vi "stringtoxml.vi"(1 "String to write":string, 2 "XML Tag":string) -> (0 "xml string":string)   [LabVIEW 2012]
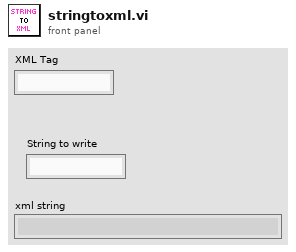
[diagram p1: front panel]
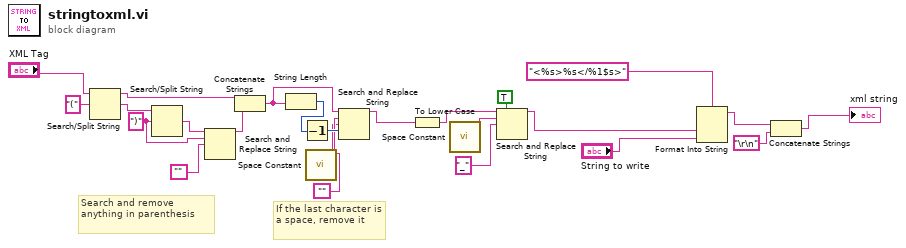
[diagram p0: block diagram]
diagram:
  w9 = ")" ("search string/char (-)")
  # "If the last character is a space, remove it"
  # "Search and remove anything in parenthesis"
  n1 = Search/Split String(string="XML Tag", search string/char (-)="(") -> (substring before match=w12:string, match + rest of string=w13:string)  [unwired: 1 in, 1 out]
  n2 = Search/Split String(string=w13, search string/char (-)=w9) -> (match + rest of string=w11:string)  [unwired: 1 in, 2 out]
  n3 = Search and Replace String(input string=w11, search string=w9, replace string="") -> (result string=w8:string)  [unwired: 5 in, 3 out]
  n4 = Concatenate Strings(w12, w8) -> (w5:string)
  n5 = String Length(string=w5) -> (length=w7:i32)
  n6 = Decrement(x=w7) -> (x-1=w6:i32)
  n7 = call <vilib>:"Space Constant.vi"() -> ("String"=w4:string)
  n8 = Search and Replace String(input string=w5, search string=w4, replace string="", offset=w6) -> (result string=w1:string)  [unwired: 4 in, 3 out]
  n9 = To Lower Case(string=w1) -> (all lower case string=w19:string)
  n10 = call <vilib>:"Space Constant.vi"() -> ("String"=w17:string)
  n11 = Search and Replace String(replace all?=TRUE ("replace all? (F)"), input string=w19, search string=w17, replace string="_") -> (result string=w15:string)  [unwired: 4 in, 3 out]
  n12 = Format Into String(format string="<%s>%s</%1$s>" ("format string (<%s>%d</%1$s>)"), w15, "String to write") -> (resulting string=w22:string)  [unwired: 2 in, 1 out]
  n13 = Concatenate Strings(w22, "\r\n") -> (→"xml string":string)
